vi "Tank height conversion.vi"() -> (2 "Height Array":dbl[](array[numeric]))   [LabVIEW 2011]
uses:
  Pumps_Valves_Dependencies_Global.vi
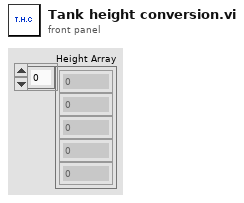
[diagram p1: front panel]
types:
  T1 = cluster{"[0]":dbl, "[1]":dbl, "[2]":dbl, "[3]":dbl, "[4]":dbl}
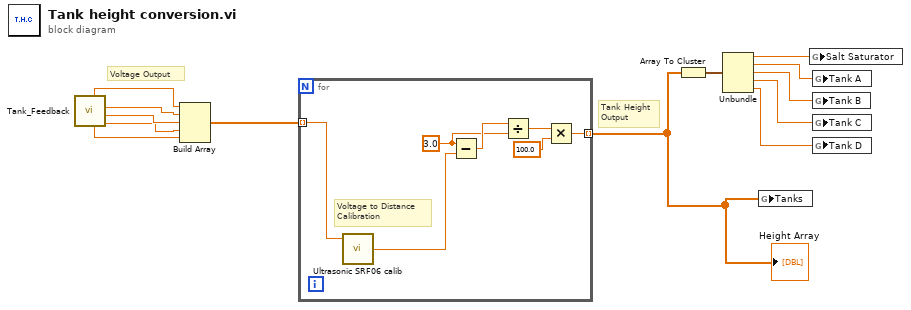
[diagram p0: block diagram]
diagram:
  # "Tank Height\nOutput"
  # "Voltage Output"
  n1 = call "Tank_Feedback.vi"() -> ("Tank D Level"=w10:dbl, "Salt Saturator Level"=w8:dbl, "Tank C Level"=w11:dbl, "Tank B Level"=w12:dbl, "Tank A Level"=w13:dbl)  [unwired: 3 in, 2 out]
  n2 = Build Array(w8, w13, w12, w11, w10) -> (w9:dbl[])
  n3 = for {
    tunnel: w9 -> [w20] mode=indexing
    tunnel: [w14] -> w7 mode=indexing
    w17 = 3.0 ("x")
    # "Voltage to Distance\nCalibration"
    n4 = call "Ultrasonic SRF06 calib.vi"("Sensor Voltage (V)"=w20) -> ("Distance (m)"=w19:dbl)  [unwired: 2 in]
    n5 = Subtract(x=w17, y=w19) -> (x-y=w18:dbl)
    n6 = Divide(x=w18, y=w17) -> (x/y=w16:dbl)
    n7 = Multiply(x=w16, y=100.0) -> (x*y=w14:dbl)
  }
  "Height Array" <- w7
  n8 = Array To Cluster(array=w7) -> (cluster=w6:T1)
  n9 = Unbundle(w6) -> ("[0]"=w5:dbl, "[1]"=w4:dbl, "[2]"=w3:dbl, "[3]"=w2:dbl, "[4]"=w1:dbl)
  n10 = global write "Pumps_Valves_Dependencies_Global.vi" "Tanks"(w7) -> ()
  n11 = global write "Pumps_Valves_Dependencies_Global.vi" "Salt Saturator"(w5) -> ()
  n12 = global write "Pumps_Valves_Dependencies_Global.vi" "Tank A"(w4) -> ()
  n13 = global write "Pumps_Valves_Dependencies_Global.vi" "Tank B"(w3) -> ()
  n14 = global write "Pumps_Valves_Dependencies_Global.vi" "Tank C"(w2) -> ()
  n15 = global write "Pumps_Valves_Dependencies_Global.vi" "Tank D"(w1) -> ()
